vi "Build.vi"(8 "error in (no error)":errorcluster, 10 "Pizza":refnum<class "Pizza(Product).lvclass">, 11 "PizzaBuilder(Builder) in":refnum<class "PizzaBuilder(Builder).lvclass">) -> (0 "error out":errorcluster, 2 "Pizza out":refnum<class "Pizza(Product).lvclass">, 3 "PizzaBuilder(Builder) out":refnum<class "PizzaBuilder(Builder).lvclass">)   [LabVIEW 2014, in "PizzaBuilder(Builder).lvclass"]
uses:
  PizzaBuilder(Builder).lvclass
  Pizza(Product)/Pizza(Product).lvclass
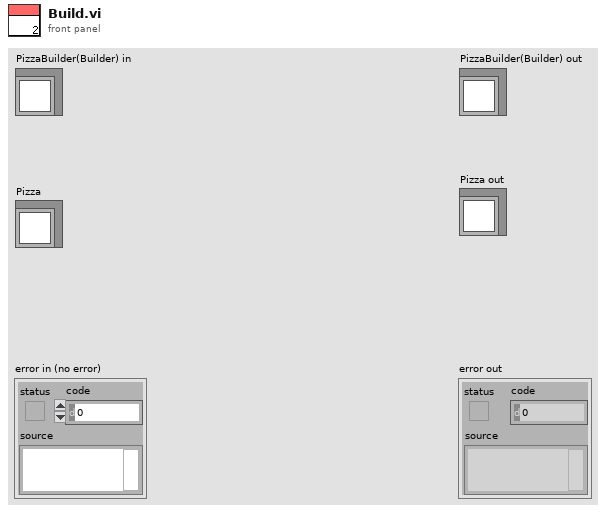
[diagram p1: front panel]
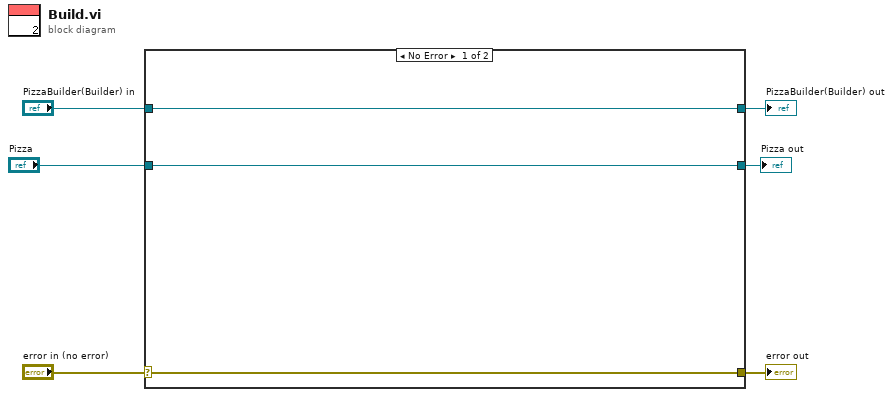
[diagram p0: block diagram]
diagram:
  n1 = case shown="No Error" "error in (no error)" {
    selector: "error in (no error)" -> [w8 w12]
    tunnel: [w8 w12] -> w5
    tunnel: [w9 w11] -> w3
    tunnel: "PizzaBuilder(Builder) in" -> [w9 w11]
    tunnel: [w7 w10] -> w2
    tunnel: "Pizza" -> [w7 w10]
    frame No Error {
    }
    frame Error {
    }
  }
  "error out" <- w5
  "PizzaBuilder(Builder) out" <- w3
  "Pizza out" <- w2
